vi "New_Magazine_Hardware_Globals.vi"() -> ()   [LabVIEW 2019]
panel:
  in  "New_Magazine_Motor_A":string
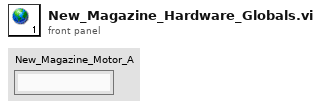
[diagram p1: front panel]
diagram:
